vi "nanocal -- nuclear schottky fit V8.vi"() -> ()   [LabVIEW 2021] (continued)
  ,  \"σlogτN\" -> 0.000000000000   ,  \"σητ1\" -> 0.000000000000   ,  \"σητS \" -> 0.000000000000   ,  \"σητN\" -> 0.000000000000    |>   , \r\"IDS0413_220525_RAW_cal__sam_\" ->   <|    \"ζ\" -> 0.044690907244   ,  \"τ1\" -> 0.013320614253   ,  \"τS\" -> 0.013760942515   ,  \"τN\" -> 0.002327045716   ,  \"τC\" -> 0.001523256988   ,  \"κ0\" -> 0.000000001960   ,  \"mm1\" -> 0.000059136229   ,  \"mm2\" -> 0.009591413737   ,  \"mm3\" -> 0.022000296296   ,  \"T\" -> 0.360000000000   ,  \"B\" -> 0.000000000000   ,  \"θ\" -> 0.000000000000   ,  \"Reoff\" -> -7142857.142857141800   ,  \"Imoff\" -> 0.000000000000   ,  \"στ1\" -> 0.002601583253   ,  \"στS\" -> 0.000378567326   ,  \"στN\" -> 0.000355149378   ,  \"τ11 \" -> 0.000000000000   ,  \"τ12\" -> 0.000000000000   ,  \"τ22\" -> 0.000000000000   ,  \"τN1\" -> 0.000000000000   ,  \"τN2\" -> 0.000000000000   ,  \"σηlogτ1 \" -> 0.000000000000   ,  \"σηlogτS\" -> 0.000000000000   ,  \"σηlogτN\" -> 0.000000000000   ,  \"σlogτ1\" -> 0.000000000000   ,  \"σlogτS\" -> 0.000000000000   ,  \"σlogτN\" -> 0.000000000000   ,  \"σητ1\" -> 0.000000000000   ,  \"σητS \" -> 0.000000000000   ,  \"σητN\" -> 0.000000000000    |>   , \r\"IDS0414_220525_RAW_cal__ref_\" ->   <|    \"ζ\" -> 0.062609276926   ,  \"τ1\" -> 0.008775091045   ,  \"τS\" -> 0.010532925062   ,  \"τN\" -> 0.001963246111   ,  \"τC\" -> 0.001185562237   ,  \"κ0\" -> 0.000000002220   ,  \"mm1\" -> 0.000063480840   ,  \"mm2\" -> 0.006468821738   ,  \"mm3\" -> 0.016706898118   ,  \"T\" -> 0.430000000000   ,  \"B\" -> 0.000000000000   ,  \"θ\" -> 0.000000000000   ,  \"Reoff\" -> -7657142.857142858210   ,  \"Imoff\" -> 0.000000000000   ,  \"στ1\" -> 0.001587412963   ,  \"στS\" -> 0.001748149515   ,  \"στN\" -> 0.000451539809   ,  \"τ11 \" -> 0.000000000000   ,  \"τ12\" -> 0.000000000000   ,  \"τ22\" -> 0.000000000000   ,  \"τN1\" -> 0.000000000000   ,  \"τN2\" -> 0.000000000000   ,  \"σηlogτ1 \" -> 0.000000000000   ,  \"σηlogτS\" -> 0.000000000000   ,  \"σηlogτN\" -> 0.000000000000   ,  \"σlogτ1\" -> 0.000000000000   ,  \"σlogτS\" -> 0.000000000000   ,  \"σlogτN\" -> 0.000000000000   ,  \"σητ1\" -> 0.000000000000   ,  \"σητS \" -> 0.000000000000   ,  \"σητN\" -> 0.000000000000    |>   , \r\"IDS0414_220525_RAW_cal__sam_\" ->   <|    \"ζ\" -> 0.036206503728   ,  \"τ1\" -> 0.010323598347   ,  \"τS\" -> 0.013793333734   ,  \"τN\" -> 0.001947462554   ,  \"τC\" -> 0.001576858934   ,  \"κ0\" -> 0.000000002450   ,  \"mm1\" -> 0.000049775806   ,  \"mm2\" -> 0.008169881573   ,  \"mm3\" -> 0.019991515390   ,  \"T\" -> 0.430000000000   ,  \"B\" -> 0.000000000000   ,  \"θ\" -> 0.000000000000   ,  \"Reoff\" -> -5183673.469387754800   ,  \"Imoff\" -> 0.000000000000   ,  \"στ1\" -> 0.000547128250   ,  \"στS\" -> 0.000218959699   ,  \"στN\" -> 0.000102085685   ,  \"τ11 \" -> 0.000000000000   ,  \"τ12\" -> 0.000000000000   ,  \"τ22\" -> 0.000000000000   ,  \"τN1\" -> 0.000000000000   ,  \"τN2\" -> 0.000000000000   ,  \"σηlogτ1 \" -> 0.000000000000   ,  \"σηlogτS\" -> 0.000000000000   ,  \"σηlogτN\" -> 0.000000000000   ,  \"σlogτ1\" -> 0.000000000000   ,  \"σlogτS\" -> 0.000000000000   ,  \"σlogτN\" -> 0.000000000000   ,  \"σητ1\" -> 0.000000000000   ,  \"σητS \" -> 0.000000000000   ,  \"σητN\" -> 0.000000000000    |>   , \r\"IDS0415_220525_RAW_cal__ref_\" ->   <|    \"ζ\" -> 0.048185231284   ,  \"τ1\" -> 0.008100929282   ,  \"τS\" -> 0.011138600782   ,  \"τN\" -> 0.001553114505   ,  \"τC\" -> 0.001221442635   ,  \"κ0\" -> 0.000000002870   ,  \"mm1\" -> 0.000051029801   ,  \"mm2\" -> 0.006456930010   ,  \"mm3\" -> 0.016117680629   ,  \"T\" -> 0.530000000000   ,  \"B\" -> 0.000000000000   ,  \"θ\" -> 0.000000000000   ,  \"Reoff\" -> -5600000.000000000000   ,  \"Imoff\" -> 0.000000000000   ,  \"στ1\" -> 0.001291082516   ,  \"στS\" -> 0.001596793517   ,  \"στN\" -> 0.000325645365   ,  \"τ11 \" -> 0.000000000000   ,  \"τ12\" -> 0.000000000000   ,  \"τ22\" -> 0.000000000000   ,  \"τN1\" -> 0.000000000000   ,  \"τN2\" -> 0.000000000000   ,  \"σηlogτ1 \" -> 0.000000000000   ,  \"σηlogτS\" -> 0.000000000000   ,  \"σηlogτN\" -> 0.000000000000   ,  \"σlogτ1\" -> 0.000000000000   ,  \"σlogτS\" -> 0.000000000000   ,  \"σlogτN\" -> 0.000000000000   ,  \"σητ1\" -> 0.000000000000   ,  \"σητS \" -> 0.000000000000   ,  \"σητN\" -> 0.000000000000    |>   , \r\"IDS0415_220525_RAW_cal__sam_\" ->   <|    \"ζ\" -> 0.029049723552   ,  \"τ1\" -> 0.007716049820   ,  \"τS\" -> 0.014447051972   ,  \"τN\" -> 0.001246053989   ,  \"τC\" -> 0.001554051920   ,  \"κ0\" -> 0.000000003200   ,  \"mm1\" -> 0.000039813384   ,  \"mm2\" -> 0.006805314073   ,  \"mm3\" -> 0.018573960634   ,  \"T\" -> 0.530000000000   ,  \"B\" -> 0.000000000000   ,  \"θ\" -> 0.000000000000   ,  \"Reoff\" -> -3959183.673469387000   ,  \"Imoff\" -> 0.000000000000   ,  \"στ1\" -> 0.000764801064   ,  \"στS\" -> 0.002293201092   ,  \"στN\" -> 0.000221114317   ,  \"τ11 \" -> 0.000000000000   ,  \"τ12\" -> 0.000000000000   ,  \"τ22\" -> 0.000000000000   ,  \"τN1\" -> 0.000000000000   ,  \"τN2\" -> 0.000000000000   ,  \"σηlogτ1 \" -> 0.000000000000   ,  \"σηlogτS\" -> 0.000000000000   ,  \"σηlogτN\" -> 0.000000000000   ,  \"σlogτ1\" -> 0.000000000000   ,  \"σlogτS\" -> 0.000000000000   ,  \"σlogτN\" -> 0.000000000000   ,  \"σητ1\" -> 0.000000000000   ,  \"σητS \" -> 0.000000000000   ,  \"σητN\" -> 0.000000000000    |>   , \r\"IDS0416_220525_RAW_cal__ref_\" ->   <|    \"ζ\" -> 0.039880135587   ,  \"τ1\" -> 0.006886163932   ,  \"τS\" -> 0.012166095681   ,  \"τN\" -> 0.001127457198   ,  \"τC\" -> 0.001222704242   ,  \"κ0\" -> 0.000000003530   ,  \"mm1\" -> 0.000042889516   ,  \"mm2\" -> 0.005990891230   ,  \"mm3\" -> 0.015898788997   ,  \"T\" -> 0.630000000000   ,  \"B\" -> 0.000000000000   ,  \"θ\" -> 0.000000000000   ,  \"Reoff\" -> -4057142.857142858210   ,  \"Imoff\" -> 0.000000000000   ,  \"στ1\" -> 0.001015861741   ,  \"στS\" -> 0.001565951598   ,  \"στN\" -> 0.000225145356   ,  \"τ11 \" -> 0.000000000000   ,  \"τ12\" -> 0.000000000000   ,  \"τ22\" -> 0.000000000000   ,  \"τN1\" -> 0.000000000000   ,  \"τN2\" -> 0.000000000000   ,  \"σηlogτ1 \" -> 0.000000000000   ,  \"σηlogτS\" -> 0.000000000000   ,  \"σηlogτN\" -> 0.000000000000   ,  \"σlogτ1\" -> 0.000000000000   ,  \"σlogτS\" -> 0.000000000000   ,  \"σlogτN\" -> 0.000000000000   ,  \"σητ1\" -> 0.000000000000   ,  \"σητS \" -> 0.000000000000   ,  \"σητN\" -> 0.000000000000    |>   , \r\"IDS0416_220525_RAW_cal__sam_\" ->   <|    \"ζ\" -> 0.022998692784   ,  \"τ1\" -> 0.007393021158   ,  \"τS\" -> 0.015620230500   ,  \"τN\" -> 0.001040733682   ,  \"τC\" -> 0.001765774011   ,  \"κ0\" -> 0.000000003911   ,  \"mm1\" -> 0.000035818495   ,  \"mm2\" -> 0.006739334009   ,  \"mm3\" -> 0.019427787243   ,  \"T\" -> 0.630000000000   ,  \"B\" -> 0.000000000000   ,  \"θ\" -> 0.000000000000   ,  \"Reoff\" -> -2408163.265306121670   ,  \"Imoff\" -> 0.000000000000   ,  \"στ1\" -> 0.000980763421   ,  \"στS\" -> 0.002016923628   ,  \"στN\" -> 0.000219391445   ,  \"τ11 \" -> 0.000000000000   ,  \"τ12\" -> 0.000000000000   ,  \"τ22\" -> 0.000000000000   ,  \"τN1\" -> 0.000000000000   ,  \"τN2\" -> 0.000000000000   ,  \"σηlogτ1 \" -> 0.000000000000   ,  \"σηlogτS\" -> 0.000000000000   ,  \"σηlogτN\" -> 0.000000000000   ,  \"σlogτ1\" -> 0.000000000000   ,  \"σlogτS\" -> 0.000000000000   ,  \"σlogτN\" -> 0.000000000000   ,  \"σητ1\" -> 0.000000000000   ,  \"σητS \" -> 0.000000000000   ,  \"σητN\" -> 0.000000000000    |>   , \r\"IDS0417_220525_RAW_cal__ref_\" ->   <|    \"ζ\" -> 0.032750219175   ,  \"τ1\" -> 0.005623693280   ,  \"τS\" -> 0.015325743160   ,  \"τN\" -> 0.000717738154   ,  \"τC\" -> 0.001196295790   ,  \"κ0\" -> 0.000000004900   ,  \"mm1\" -> 0.000035343333   ,  \"mm2\" -> 0.005288786846   ,  \"mm3\" -> 0.018064767734   ,  \"T\" -> 0.830000000000   ,  \"B\" -> 0.000000000000   ,  \"θ\" -> 0.000000000000   ,  \"Reoff\" -> -3028571.428571429100   ,  \"Imoff\" -> 0.000000000000   ,  \"στ1\" -> 0.003777268036   ,  \"στS\" -> 0.001674973783   ,  \"στN\" -> 0.000298996570   ,  \"τ11 \" -> 0.000000000000   ,  \"τ12\" -> 0.000000000000   ,  \"τ22\" -> 0.000000000000   ,  \"τN1\" -> 0.000000000000   ,  \"τN2\" -> 0.000000000000   ,  \"σηlogτ1 \" -> 0.000000000000   ,  \"σηlogτS\" -> 0.000000000000   ,  \"σηlogτN\" -> 0.000000000000   ,  \"σlogτ1\" -> 0.000000000000   ,  \"σlogτS\" -> 0.000000000000   ,  \"σlogτN\" -> 0.000000000000   ,  \"σητ1\" -> 0.000000000000   ,  \"σητS \" -> 0.000000000000   ,  \"σητN\" -> 0.000000000000    |>   , \r\"IDS0417_220525_RAW_cal__sam_\" ->   <|    \"ζ\" -> 0.020422056832   ,  \"τ1\" -> 0.006457484957   ,  \"τS\" -> 0.019722165301   ,  \"τN\" -> 0.000729413719   ,  \"τC\" -> 0.001622930071   ,  \"κ0\" -> 0.000000005380   ,  \"mm1\" -> 0.000030097695   ,  \"mm2\" -> 0.006162713408   ,  \"mm3\" -> 0.022756846254   ,  \"T\" -> 0.830000000000   ,  \"B\" -> 0.000000000000   ,  \"θ\" -> 0.000000000000   ,  \"Reoff\" -> -2081632.653061224150   ,  \"Imoff\" -> 0.000000000000   ,  \"στ1\" -> 0.000977899540   ,  \"στS\" -> 0.002370947727   ,  \"στN\" -> 0.000160479256   ,  \"τ11 \" -> 0.000000000000   ,  \"τ12\" -> 0.000000000000   ,  \"τ22\" -> 0.000000000000   ,  \"τN1\" -> 0.000000000000   ,  \"τN2\" -> 0.000000000000   ,  \"σηlogτ1 \" -> 0.000000000000   ,  \"σηlogτS\" -> 0.000000000000   ,  \"σηlogτN\" -> 0.000000000000   ,  \"σlogτ1\" -> 0.000000000000   ,  \"σlogτS\" -> 0.000000000000   ,  \"σlogτN\" -> 0.000000000000   ,  \"σητ1\" -> 0.000000000000   ,  \"σητS \" -> 0.000000000000   ,  \"σητN\" -> 0.000000000000    |>   , \r\"IDS0418_220525_RAW_cal__ref_\" ->   <|    \"ζ\" -> 0.022904137166   ,  \"τ1\" -> 0.004842430213   ,  \"τS\" -> 0.021231337399   ,  \"τN\" -> 0.000595878691   ,  \"τC\" -> 0.001701256533   ,  \"κ0\" -> 0.000000006850   ,  \"mm1\" -> 0.000035378969   ,  \"mm2\" -> 0.004689611444   ,  \"mm3\" -> 0.024145845974   ,  \"T\" -> 1.120000000000   ,  \"B\" -> 0.000000000000   ,  \"θ\" -> 0.000000000000   ,  \"Reoff\" -> -1314285.714285716420   ,  \"Imoff\" -> 0.000000000000   ,  \"στ1\" -> 0.000594455147   ,  \"στS\" -> 0.001847173468   ,  \"στN\" -> 0.000101337306   ,  \"τ11 \" -> 0.000000000000   ,  \"τ12\" -> 0.000000000000   ,  \"τ22\" -> 0.000000000000   ,  \"τN1\" -> 0.000000000000   ,  \"τN2\" -> 0.000000000000   ,  \"σηlogτ1 \" -> 0.000000000000   ,  \"σηlogτS\" -> 0.000000000000   ,  \"σηlogτN\" -> 0.000000000000   ,  \"σlogτ1\" -> 0.000000000000   ,  \"σlogτS\" -> 0.000000000000   ,  \"σlogτN\" -> 0.000000000000   ,  \"σητ1\" -> 0.000000000000   ,  \"σητS \" -> 0.000000000000   ,  \"σητN\" -> 0.000000000000    |>   , \r\"IDS0418_220525_RAW_cal__sam_\" ->   <|    \"ζ\" -> 0.010833914814   ,  \"τ1\" -> 0.006105280968   ,  \"τS\" -> 0.027771405990   ,  \"τN\" -> 0.000655710517   ,  \"τC\" -> 0.001898693697   ,  \"κ0\" -> 0.000000007420   ,  \"mm1\" -> 0.000019072683   ,  \"mm2\" -> 0.005941306089   ,  \"mm3\" -> 0.030778689359   ,  \"T\" -> 1.120000000000   ,  \"B\" -> 0.000000000000   ,  \"θ\" -> 0.000000000000   ,  \"Reoff\" -> -608163.265306122367   ,  \"Imoff\" -> 0.000000000000   ,  \"στ1\" -> 0.001326459237   ,  \"στS\" -> 0.003728359065   ,  \"στN\" -> 0.000181682896   ,  \"τ11 \" -> 0.000000000000   ,  \"τ12\" -> 0.000000000000   ,  \"τ22\" -> 0.000000000000   ,  \"τN1\" -> 0.000000000000   ,  \"τN2\" -> 0.000000000000   ,  \"σηlogτ1 \" -> 0.000000000000   ,  \"σηlogτS\" -> 0.000000000000   ,  \"σηlogτN\" -> 0.000000000000   ,  \"σlogτ1\" -> 0.000000000000   ,  \"σlogτS\" -> 0.000000000000   ,  \"σlogτN\" -> 0.000000000000   ,  \"σητ1\" -> 0.000000000000   ,  \"σητS \" -> 0.000000000000   ,  \"σητN\" -> 0.000000000000    |>   , \r\"IDS0419_220525_RAW_cal__ref_\" ->   <|    \"ζ\" -> 0.019588015905   ,  \"τ1\" -> 0.004781626559   ,  \"τS\" -> 0.047742438651   ,  \"τN\" -> 0.000600848305   ,  \"τC\" -> 0.002316865749   ,  \"κ0\" -> 0.000000012200   ,  \"mm1\" -> 0.000042523875   ,  \"mm2\" -> 0.004719121437   ,  \"mm3\" -> 0.051627083026   ,  \"T\" -> 1.900000000000   ,  \"B\" -> 0.000000000000   ,  \"θ\" -> 0.000000000000   ,  \"Reoff\" -> -714285.714285716413   ,  \"Imoff\" -> 0.000000000000   ,  \"στ1\" -> 0.001059318885   ,  \"στS\" -> 0.005613918235   ,  \"στN\" -> 0.000174681152   ,  \"τ11 \" -> 0.000000000000   ,  \"τ12\" -> 0.000000000000   ,  \"τ22\" -> 0.000000000000   ,  \"τN1\" -> 0.000000000000   ,  \"τN2\" -> 0.000000000000   ,  \"σηlogτ1 \" -> 0.000000000000   ,  \"σηlogτS\" -> 0.000000000000   ,  \"σηlogτN\" -> 0.000000000000   ,  \"σlogτ1\" -> 0.000000000000   ,  \"σlogτS\" -> 0.000000000000   ,  \"σlogτN\" -> 0.000000000000   ,  \"σητ1\" -> 0.000000000000   ,  \"σητS \" -> 0.000000000000   ,  \"σητN\" -> 0.000000000000    |>   , \r\"IDS0419_220525_RAW_cal__sam_\" ->   <|    \"ζ\" -> 0.011595776290   ,  \"τ1\" -> 0.006117918264   ,  \"τS\" -> 0.061916055974   ,  \"τN\" -> 0.000669101537   ,  \"τC\" -> 0.002022450323   ,  \"κ0\" -> 0.000000012950   ,  \"mm1\" -> 0.000022465670   ,  \"mm2\" -> 0.006048051710   ,  \"mm3\" -> 0.065380732203   ,  \"T\" -> 1.900000000000   ,  \"B\" -> 0.000000000000   ,  \"θ\" -> 0.000000000000   ,  \"Reoff\" -> -608163.265306122367   ,  \"Imoff\" -> 0.000000000000   ,  \"στ1\" -> 0.001547930555   ,  \"στS\" -> 0.007827805463   ,  \"στN\" -> 0.000227173092   ,  \"τ11 \" -> 0.000000000000   ,  \"τ12\" -> 0.000000000000   ,  \"τ22\" -> 0.000000000000   ,  \"τN1\" -> 0.000000000000   ,  \"τN2\" -> 0.000000000000   ,  \"σηlogτ1 \" -> 0.000000000000   ,  \"σηlogτS\" -> 0.000000000000   ,  \"σηlogτN\" -> 0.000000000000   ,  \"σlogτ1\" -> 0.000000000000   ,  \"σlogτS\" -> 0.000000000000   ,  \"σlogτN\" -> 0.000000000000   ,  \"σητ1\" -> 0.000000000000   ,  \"σητS \" -> 0.000000000000   ,  \"σητN\" -> 0.000000000000    |>   , \r\"IDS0420_220525_RAW_cal__ref_\" ->   <|    \"ζ\" -> 0.020834428044   ,  \"τ1\" -> 0.004699063518   ,  \"τS\" -> 0.052089260804   ,  \"τN\" -> 0.000594934592   ,  \"τC\" -> 0.002174562230   ,  \"κ0\" -> 0.000000013800   ,  \"mm1\" -> 0.000042670178   ,  \"mm2\" -> 0.004643420551   ,  \"mm3\" -> 0.055969375493   ,  \"T\" -> 2.100000000000   ,  \"B\" -> 0.000000000000   ,  \"θ\" -> 0.000000000000   ,  \"Reoff\" -> -714285.714285716413   ,  \"Imoff\" -> 0.000000000000   ,  \"στ1\" -> 0.001320131062   ,  \"στS\" -> 0.004774189877   ,  \"στN\" -> 0.000170930701   ,  \"τ11 \" -> 0.000000000000   ,  \"τ12\" -> 0.000000000000   ,  \"τ22\" -> 0.000000000000   ,  \"τN1\" -> 0.000000000000   ,  \"τN2\" -> 0.000000000000   ,  \"σηlogτ1 \" -> 0.000000000000   ,  \"σηlogτS\" -> 0.000000000000   ,  \"σηlogτN\" -> 0.000000000000   ,  \"σlogτ1\" -> 0.000000000000   ,  \"σlogτS\" -> 0.000000000000   ,  \"σlogτN\" -> 0.000000000000   ,  \"σητ1\" -> 0.000000000000   ,  \"σητS \" -> 0.000000000000   ,  \"σητN\" -> 0.000000000000    |>   , \r\"IDS0420_220525_RAW_cal__sam_\" ->   <|    \"ζ\" -> 0.011850996022   ,  \"τ1\" -> 0.005764384736   ,  \"τS\" -> 0.066220067505   ,  \"τN\" -> 0.000645440877   ,  \"τC\" -> 0.002901198812   ,  \"κ0\" -> 0.000000014700   ,  \"mm1\" -> 0.000032584327   ,  \"mm2\" -> 0.005706320364   ,  \"mm3\" -> 0.070584610113   ,  \"T\" -> 2.100000000000   ,  \"B\" -> 0.000000000000   ,  \"θ\" -> 0.000000000000   ,  \"Reoff\" -> -461224.489795918343   ,  \"Imoff\" -> 0.000000000000   ,  \"στ1\" -> 0.000879947943   ,  \"στS\" -> 0.005816006372   ,  \"στN\" -> 0.000150645668   ,  \"τ11 \" -> 0.000000000000   ,  \"τ12\" -> 0.000000000000   ,  \"τ22\" -> 0.000000000000   ,  \"τN1\" -> 0.000000000000   ,  \"τN2\" -> 0.000000000000   ,  \"σηlogτ1 \" -> 0.000000000000   ,  \"σηlogτS\" -> 0.000000000000   ,  \"σηlogτN\" -> 0.000000000000   ,  \"σlogτ1\" -> 0.000000000000   ,  \"σlogτS\" -> 0.000000000000   ,  \"σlogτN\" -> 0.000000000000   ,  \"σητ1\" -> 0.000000000000   ,  \"σητS \" -> 0.000000000000   ,  \"σητN\" -> 0.000000000000    |>   , \r\"IDS0421_220525_RAW_cal__ref_\" ->   <|    \"ζ\" -> 0.022335092396   ,  \"τ1\" -> 0.004357676744   ,  \"τS\" -> 0.014734142286   ,  \"τN\" -> 0.000494755663   ,  \"τC\" -> 0.002291218216   ,  \"κ0\" -> 0.000000015200   ,  \"mm1\" -> 0.000043555244   ,  \"mm2\" -> 0.004196096690   ,  \"mm3\" -> 0.017978279817   ,  \"T\" -> 2.300000000000   ,  \"B\" -> 0.000000000000   ,  \"θ\" -> 0.000000000000   ,  \"Reoff\" -> -714285.714285716413   ,  \"Imoff\" -> 0.000000000000   ,  \"στ1\" -> 0.001017327919   ,  \"στS\" -> 0.002314643379   ,  \"στN\" -> 0.000146182526   ,  \"τ11 \" -> 0.000000000000   ,  \"τ12\" -> 0.000000000000   ,  \"τ22\" -> 0.000000000000   ,  \"τN1\" -> 0.000000000000   ,  \"τN2\" -> 0.000000000000   ,  \"σηlogτ1 \" -> 0.000000000000   ,  \"σηlogτS\" -> 0.000000000000   ,  \"σηlogτN\" -> 0.000000000000   ,  \"σlogτ1\" -> 0.000000000000   ,  \"σlogτS\" -> 0.000000000000   ,  \"σlogτN\" -> 0.000000000000   ,  \"σητ1\" -> 0.000000000000   ,  \"σητS \" -> 0.000000000000   ,  \"σητN\" -> 0.000000000000    |>   , \r\"IDS0421_220525_RAW_cal__sam_\" ->   <|    \"ζ\" -> 0.017472306497   ,  \"τ1\" -> 0.005884707777   ,  \"τS\" -> 0.018273540555   ,  \"τN\" -> 0.000393530305   ,  \"τC\" -> 0.002873982576   ,  \"κ0\" -> 0.000000016000   ,  \"mm1\" -> 0.000042829990   ,  \"mm2\" -> 0.005738391469   ,  \"mm3\" -> 0.021970696537   ,  \"T\" -> 2.300000000000   ,  \"B\" -> 0.000000000000   ,  \"θ\" -> 0.000000000000   ,  \"Reoff\" -> -616326.530612244968   ,  \"Imoff\" -> 0.000000000000   ,  \"στ1\" -> 0.001449504442   ,  \"στS\" -> 0.003094967894   ,  \"στN\" -> 0.000132016087   ,  \"τ11 \" -> 0.000000000000   ,  \"τ12\" -> 0.000000000000   ,  \"τ22\" -> 0.000000000000   ,  \"τN1\" -> 0.000000000000   ,  \"τN2\" -> 0.000000000000   ,  \"σηlogτ1 \" -> 0.000000000000   ,  \"σηlogτS\" -> 0.000000000000   ,  \"σηlogτN\" -> 0.000000000000   ,  \"σlogτ1\" -> 0.000000000000   ,  \"σlogτS\" -> 0.000000000000   ,  \"σlogτN\" -> 0.000000000000   ,  \"σητ1\" -> 0.000000000000   ,  \"σητS \" -> 0.000000000000   ,  \"σητN\" -> 0.000000000000    |>   , \r\"IDS0422_220525_RAW_cal__ref_\" ->   <|    \"ζ\" -> 0.018555902016   ,  \"τ1\" -> 0.004075291246   ,  \"τS\" -> 0.009145270052   ,  \"τN\" -> 0.000208864759   ,  \"τC\" -> 0.002022167505   ,  \"κ0\" -> 0.000000022500   ,  \"mm1\" -> 0.000030348931   ,  \"mm2\" -> 0.003960776557   ,  \"mm3\" -> 0.011634042483   ,  \"T\" -> 3.100000000000   ,  \"B\" -> 0.000000000000   ,  \"θ\" -> 0.000000000000   ,  \"Reoff\" -> -371428.571428570896   ,  \"Imoff\" -> 0.000000000000   ,  \"στ1\" -> 0.000657121780   ,  \"στS\" -> 0.001216403398   ,  \"στN\" -> 0.000050486757   ,  \"τ11 \" -> 0.000000000000   ,  \"τ12\" -> 0.000000000000   ,  \"τ22\" -> 0.000000000000   ,  \"τN1\" -> 0.000000000000   ,  \"τN2\" -> 0.000000000000   ,  \"σηlogτ1 \" -> 0.000000000000   ,  \"σηlogτS\" -> 0.000000000000   ,  \"σηlogτN\" -> 0.000000000000   ,  \"σlogτ1\" -> 0.000000000000   ,  \"σlogτS\" -> 0.000000000000   ,  \"σlogτN\" -> 0.000000000000   ,  \"σητ1\" -> 0.000000000000   ,  \"σητS \" -> 0.000000000000   ,  \"σητN\" -> 0.000000000000    |>   , \r\"IDS0422_220525_RAW_cal__sam_\" ->   <|    \"ζ\" -> 0.013782660001   ,  \"τ1\" -> 0.005602489845   ,  \"τS\" -> 0.011122141420   ,  \"τN\" -> 0.000341635093   ,  \"τC\" -> 0.002887063483   ,  \"κ0\" -> 0.000000023500   ,  \"mm1\" -> 0.000031317292   ,  \"mm2\" -> 0.005389288482   ,  \"mm3\" -> 0.014690725401   ,  \"T\" -> 3.100000000000   ,  \"B\" -> 0.000000000000   ,  \"θ\" -> 0.000000000000   ,  \"Reoff\" -> -338775.510204081656   ,  \"Imoff\" -> 0.000000000000   ,  \"στ1\" -> 0.000787586702   ,  \"στS\" -> 0.001319427978   ,  \"στN\" -> 0.000072408344   ,  \"τ11 \" -> 0.000000000000   ,  \"τ12\" -> 0.000000000000   ,  \"τ22\" -> 0.000000000000   ,  \"τN1\" -> 0.000000000000   ,  \"τN2\" -> 0.000000000000   ,  \"σηlogτ1 \" -> 0.000000000000   ,  \"σηlogτS\" -> 0.000000000000   ,  \"σηlogτN\" -> 0.000000000000   ,  \"σlogτ1\" -> 0.000000000000   ,  \"σlogτS\" -> 0.000000000000   ,  \"σlogτN\" -> 0.000000000000   ,  \"σητ1\" -> 0.000000000000   ,  \"σητS \" -> 0.000000000000   ,  \"σητN\" -> 0.000000000000    |>   , \r\"IDS0424_220526_RAW_cal__ref_\" ->   <|    \"ζ\" -> 0.257512497689   ,  \"τ1\" -> 0.039924767980   ,  \"τS\" -> 0.063776955906   ,  \"τN\" -> 0.051107290948   ,  \"τC\" -> 0.000802475621   ,  \"κ0\" -> 0.000000000773   ,  \"mm1\" -> 0.000163026258   ,  \"mm2\" -> 0.019497997616   ,  \"mm3\" -> 0.165534595934   ,  \"T\" -> 0.190000000000   ,  \"B\" -> 10.000000000000   ,  \"θ\" -> 0.000000000000   ,  \"Reoff\" -> -55142857.142857134400   ,  \"Imoff\" -> 0.000000000000   ,  \"στ1\" -> 0.000058307175   ,  \"στS\" -> 0.000031998048   ,  \"στN\" -> 0.000036682192   ,  \"τ11 \" -> 0.000000000000   ,  \"τ12\" -> 0.000000000000   ,  \"τ22\" -> 0.000000000000   ,  \"τN1\" -> 0.000000000000   ,  \"τN2\" -> 0.000000000000   ,  \"σηlogτ1 \" -> 0.000000000000   ,  \"σηlogτS\" -> 0.000000000000   ,  \"σηlogτN\" -> 0.000000000000   ,  \"σlogτ1\" -> 0.000000000000   ,  \"σlogτS\" -> 0.000000000000   ,  \"σlogτN\" -> 0.000000000000   ,  \"σητ1\" -> 0.000000000000   ,  \"σητS \" -> 0.000000000000   ,  \"σητN\" -> 0.000000000000    |>   , \r\"IDS0424_220526_RAW_cal__sam_\" ->   <|    \"ζ\" -> 0.143096873941   ,  \"τ1\" -> 0.119527741552   ,  \"τS\" -> 0.213771204505   ,  \"τN\" -> 0.133065206622   ,  \"τC\" -> 0.001041786526   ,  \"κ0\" -> 0.000000000890   ,  \"mm1\" -> 0.000129929317   ,  \"mm2\" -> 0.064852834373   ,  \"mm3\" -> 0.452054381716   ,  \"T\" -> 0.190000000000   ,  \"B\" -> 10.000000000000   ,  \"θ\" -> 0.000000000000   ,  \"Reoff\" -> -41461224.489795915800   ,  \"Imoff\" -> 0.000000000000   ,  \"στ1\" -> 0.142328196867   ,  \"στS\" -> 0.153709890516   ,  \"στN\" -> 0.034979737706   ,  \"τ11 \" -> 0.000000000000   ,  \"τ12\" -> 0.000000000000   ,  \"τ22\" -> 0.000000000000   ,  \"τN1\" -> 0.000000000000   ,  \"τN2\" -> 0.000000000000   ,  \"σηlogτ1 \" -> 0.000000000000   ,  \"σηlogτS\" -> 0.000000000000   ,  \"σηlogτN\" -> 0.000000000000   ,  \"σlogτ1\" -> 0.000000000000   ,  \"σlogτS\" -> 0.000000000000   ,  \"σlogτN\" -> 0.000000000000   ,  \"σητ1\" -> 0.000000000000   ,  \"σητS \" -> 0.000000000000   ,  \"σητN\" -> 0.000000000000    |>   , \r\"IDS0425_220526_RAW_cal__ref_\" ->   <|    \"ζ\" -> 0.159335076752   ,  \"τ1\" -> 0.031885685275   ,  \"τS\" -> 0.047996731633   ,  \"τN\" -> 0.019207310502   ,  \"τC\" -> 0.000887935907   ,  \"κ0\" -> 0.000000001118   ,  \"mm1\" -> 0.000120371950   ,  \"mm2\" -> 0.019822778110   ,  \"mm3\" -> 0.090742474469   ,  \"T\" -> 0.250000000000   ,  \"B\" -> 10.000000000000   ,  \"θ\" -> 0.000000000000   ,  \"Reoff\" -> -27579558.011049721400   ,  \"Imoff\" -> 0.000000000000   ,  \"στ1\" -> 0.000105033309   ,  \"στS\" -> 0.000027614157   ,  \"στN\" -> 0.000060474658   ,  \"τ11 \" -> 0.000000000000   ,  \"τ12\" -> 0.000000000000   ,  \"τ22\" -> 0.000000000000   ,  \"τN1\" -> 0.000000000000   ,  \"τN2\" -> 0.000000000000   ,  \"σηlogτ1 \" -> 0.000000000000   ,  \"σηlogτS\" -> 0.000000000000   ,  \"σηlogτN\" -> 0.000000000000   ,  \"σlogτ1\" -> 0.000000000000   ,  \"σlogτS\" -> 0.000000000000   ,  \"σlogτN\" -> 0.000000000000   ,  \"σητ1\" -> 0.000000000000   ,  \"σητS \" -> 0.000000000000   ,  \"σητN\" -> 0.000000000000    |>   , \r\"IDS0425_220526_RAW_cal__sam_\" ->   <|    \"ζ\" -> 0.080613368975   ,  \"τ1\" -> 0.039981630615   ,  \"τS\" -> 0.067451052819   ,  \"τN\" -> 0.024952731947   ,  \"τC\" -> 0.001301901326   ,  \"κ0\" -> 0.000000001270   ,  \"mm1\" -> 0.000095538727   ,  \"mm2\" -> 0.025680137218   ,  \"mm3\" -> 0.115360621158   ,  \"T\" -> 0.250000000000   ,  \"B\" -> 10.000000000000   ,  \"θ\" -> 0.000000000000   ,  \"Reoff\" -> -15077551.020408168400   ,  \"Imoff\" -> 0.000000000000   ,  \"στ1\" -> 0.017921325903   ,  \"στS\" -> 0.008554959302   ,  \"στN\" -> 0.012696106226   ,  \"τ11 \" -> 0.000000000000   ,  \"τ12\" -> 0.000000000000   ,  \"τ22\" -> 0.000000000000   ,  \"τN1\" -> 0.000000000000   ,  \"τN2\" -> 0.000000000000   ,  \"σηlogτ1 \" -> 0.000000000000   ,  \"σηlogτS\" -> 0.000000000000   ,  \"σηlogτN\" -> 0.000000000000   ,  \"σlogτ1\" -> 0.000000000000   ,  \"σlogτS\" -> 0.000000000000   ,  \"σlogτN\" -> 0.000000000000   ,  \"σητ1\" -> 0.000000000000   ,  \"σητS \" -> 0.000000000000   ,  \"σητN\" -> 0.000000000000    |>   , \r\"IDS0426_220526_RAW_cal__ref_\" ->   <|    \"ζ\" -> 0.111460827005   ,  \"τ1\" -> 0.024224453348   ,  \"τS\" -> 0.042028783084   ,  \"τN\" -> 0.009416687783   ,  \"τC\" -> 0.001053496592   ,  \"κ0\" -> 0.000000001428   ,  \"mm1\" -> 0.000103540379   ,  \"mm2\" -> 0.017919606240   ,  \"mm3\" -> 0.064434428916   ,  \"T\" -> 0.300000000000   ,  \"B\" -> 10.000000000000   ,  \"θ\" -> 0.000000000000   ,  \"Reoff\" -> -13408163.265306122600   ,  \"Imoff\" -> 0.000000000000   ,  \"στ1\" -> 0.000203310758   ,  \"στS\" -> 0.000031022481   ,  \"στN\" -> 0.000119793909   ,  \"τ11 \" -> 0.000000000000   ,  \"τ12\" -> 0.000000000000   ,  \"τ22\" -> 0.000000000000   ,  \"τN1\" -> 0.000000000000   ,  \"τN2\" -> 0.000000000000   ,  \"σηlogτ1 \" -> 0.000000000000   ,  \"σηlogτS\" -> 0.000000000000   ,  \"σηlogτN\" -> 0.000000000000   ,  \"σlogτ1\" -> 0.000000000000   ,  \"σlogτS\" -> 0.000000000000   ,  \"σlogτN\" -> 0.000000000000   ,  \"σητ1\" -> 0.000000000000   ,  \"σητS \" -> 0.000000000000   ,  \"σητN\" -> 0.000000000000    |>   , \r\"IDS0426_220526_RAW_cal__sam_\" ->   <|    \"ζ\" -> 0.000000000000   ,  \"τ1\" -> 0.000000000000   ,  \"τS\" -> 0.000000000000   ,  \"τN\" -> 0.000000000000   ,  \"τC\" -> 0.000000000000   ,  \"κ0\" -> 0.000000000000   ,  \"mm1\" -> 0.000000000000   ,  \"mm2\" -> 0.000000000000   ,  \"mm3\" -> 0.000000000000   ,  \"T\" -> 0.300000000000   ,  \"B\" -> 10.000000000000   ,  \"θ\" -> 0.000000000000   ,  \"Reoff\" -> 0.000000000000   ,  \"Imoff\" -> 0.000000000000   ,  \"στ1\" -> 0.000000000000   ,  \"στS\" -> 0.000000000000   ,  \"στN\" -> 0.000000000000   ,  \"τ11 \" -> 0.000000000000   ,  \"τ12\" -> 0.000000000000   ,  \"τ22\" -> 0.000000000000   ,  \"τN1\" -> 0.000000000000   ,  \"τN2\" -> 0.000000000000   ,  \"σηlogτ1 \" -> 0.000000000000   ,  \"σηlogτS\" -> 0.000000000000   ,  \"σηlogτN\" -> 0.000000000000   ,  \"σlogτ1\" -> 0.000000000000   ,  \"σlogτS\" -> 0.000000000000   ,  \"σlogτN\" -> 0.000000000000   ,  \"σητ1\" -> 0.000000000000   ,  \"σητS \" -> 0.000000000000   ,  \"σητN\" -> 0.000000000000    |>   , \r\"IDS0427_220526_RAW_cal__ref_\" ->   <|    \"ζ\" -> 0.410372558234   ,  \"τ1\" -> 0.044042677076   ,  \"τS\" -> 0.102926494068   ,  \"τN\" -> 0.135379226142   ,  \"τC\" -> 0.000829804272   ,  \"κ0\" -> 0.000000000538   ,  \"mm1\" -> 0.000240462729   ,  \"mm2\" -> 0.017682403463   ,  \"mm3\" -> 0.363049463410   ,  \"T\" -> 0.150000000000   ,  \"B\" -> 10.000000000000   ,  \"θ\" -> 0.000000000000   ,  \"Reoff\" -> -106571428.571428567000   ,  \"Imoff\" -> 0.000000000000   ,  \"στ1\" -> 0.000056157157   ,  \"στS\" -> 0.000057678080   ,  \"στN\" -> 0.000041998406   ,  \"τ11 \" -> 0.000000000000   ,  \"τ12\" -> 0.000000000000   ,  \"τ22\" -> 0.000000000000   ,  \"τN1\" -> 0.000000000000   ,  \"τN2\" -> 0.000000000000   ,  \"σηlogτ1 \" -> 0.000000000000   ,  \"σηlogτS\" -> 0.000000000000   ,  \"σηlogτN\" -> 0.000000000000   ,  \"σlogτ1\" -> 0.000000000000   ,  \"σlogτS\" -> 0.000000000000   ,  \"σlogτN\" -> 0.000000000000   ,  \"σητ1\" -> 0.000000000000   ,  \"σητS \" -> 0.000000000000   ,  \"σητN\" -> 0.000000000000    |>   , \r\"IDS0427_220526_RAW_cal__sam_\" ->   <|    \"ζ\" -> 0.000000000000   ,  \"τ1\" -> 0.000000000000   ,  \"τS\" -> 0.000000000000   ,  \"τN\" -> 0.000000000000   ,  \"τC\" -> 0.000000000000   ,  \"κ0\" -> 0.000000000000   ,  \"mm1\" -> 0.000000000000   ,  \"mm2\" -> 0.000000000000   ,  \"mm3\" -> 0.000000000000   ,  \"T\" -> 0.150000000000   ,  \"B\" -> 10.000000000000   ,  \"θ\" -> 0.000000000000   ,  \"Reoff\" -> 0.000000000000   ,  \"Imoff\" -> 0.000000000000   ,  \"στ1\" -> 0.000000000000   ,  \"στS\" -> 0.000000000000   ,  \"στN\" -> 0.000000000000   ,  \"τ11 \" -> 0.000000000000   ,  \"τ12\" -> 0.000000000000   ,  \"τ22\" -> 0.000000000000   ,  \"τN1\" -> 0.000000000000   ,  \"τN2\" -> 0.000000000000   ,  \"σηlogτ1 \" -> 0.000000000000   ,  \"σηlogτS\" -> 0.000000000000   ,  \"σηlogτN\" -> 0.000000000000   ,  \"σlogτ1\" -> 0.000000000000   ,  \"σlogτS\" -> 0.000000000000   ,  \"σlogτN\" -> 0.000000000000   ,  \"σητ1\" -> 0.000000000000   ,  \"σητS \" -> 0.000000000000   ,  \"σητN\" -> 0.000000000000    |>   , \r\"IDS0428_220526_RAW_cal__ref_\" ->   <|    \"ζ\" -> 0.085761087931   ,  \"τ1\" -> 0.025055116447   ,  \"τS\" -> 0.039037181879   ,  \"τN\" -> 0.005587062279   ,  \"τC\" -> 0.001009401057   ,  \"κ0\" -> 0.000000001845   ,  \"mm1\" -> 0.000078014543   ,  \"mm2\" -> 0.019900208864   ,  \"mm3\" -> 0.054537561983   ,  \"T\" -> 0.360000000000   ,  \"B\" -> 10.000000000000   ,  \"θ\" -> 0.000000000000   ,  \"Reoff\" -> -10418232.044198893000   ,  \"Imoff\" -> 0.000000000000   ,  \"στ1\" -> 0.000347384848   ,  \"στS\" -> 0.000031989956   ,  \"στN\" -> 0.000188370043   ,  \"τ11 \" -> 0.000000000000   ,  \"τ12\" -> 0.000000000000   ,  \"τ22\" -> 0.000000000000   ,  \"τN1\" -> 0.000000000000   ,  \"τN2\" -> 0.000000000000   ,  \"σηlogτ1 \" -> 0.000000000000   ,  \"σηlogτS\" -> 0.000000000000   ,  \"σηlogτN\" -> 0.000000000000   ,  \"σlogτ1\" -> 0.000000000000   ,  \"σlogτS\" -> 0.000000000000   ,  \"σlogτN\" -> 0.000000000000   ,  \"σητ1\" -> 0.000000000000   ,  \"σητS \" -> 0.000000000000   ,  \"σητN\" -> 0.000000000000    |>   , \r\"IDS0428_220526_RAW_cal__sam_\" ->   <|    \"ζ\" -> 0.000000000000   ,  \"τ1\" -> 0.000000000000   ,  \"τS\" -> 0.000000000000   ,  \"τN\" -> 0.000000000000   ,  \"τC\" -> 0.000000000000   ,  \"κ0\" -> 0.000000000000   ,  \"mm1\" -> 0.000000000000   ,  \"mm2\" -> 0.000000000000   ,  \"mm3\" -> 0.000000000000   ,  \"T\" -> 0.360000000000   ,  \"B\" -> 10.000000000000   ,  \"θ\" -> 0.000000000000   ,  \"Reoff\" -> 0.000000000000   ,  \"Imoff\" -> 0.000000000000   ,  \"στ1\" -> 0.000000000000   ,  \"στS\" -> 0.000000000000   ,  \"στN\" -> 0.000000000000   ,  \"τ11 \" -> 0.000000000000   ,  \"τ12\" -> 0.000000000000   ,  \"τ22\" -> 0.000000000000   ,  \"τN1\" -> 0.000000000000   ,  \"τN2\" -> 0.000000000000   ,  \"σηlogτ1 \" -> 0.000000000000   ,  \"σηlogτS\" -> 0.000000000000   ,  \"σηlogτN\" -> 0.000000000000   ,  \"σlogτ1\" -> 0.000000000000   ,  \"σlogτS\" -> 0.000000000000   ,  \"σlogτN\" -> 0.000000000000   ,  \"σητ1\" -> 0.000000000000   ,  \"σητS \" -> 0.000000000000   ,  \"σητN\" -> 0.000000000000    |>   , \r\"IDS0429_220526_RAW_cal__ref_\" ->   <|    \"ζ\" -> 0.061793425944   ,  \"τ1\" -> 0.022729976964   ,  \"τS\" -> 0.037992561842   ,  \"τN\" -> 0.003473638845   ,  \"τC\" -> 0.001146343524   ,  \"κ0\" -> 0.000000002261   ,  \"mm1\" -> 0.000064971896   ,  \"mm2\" -> 0.019461604024   ,  \"mm3\" -> 0.048378283857   ,  \"T\" -> 0.420000000000   ,  \"B\" -> 10.000000000000   ,  \"θ\" -> 0.000000000000   ,  \"Reoff\" -> -5435911.602209940560   ,  \"Imoff\" -> 0.000000000000   ,  \"στ1\" -> 0.000628479456   ,  \"στS\" -> 0.000037704094   ,  \"στN\" -> 0.000344539444   ,  \"τ11 \" -> 0.000000000000   ,  \"τ12\" -> 0.000000000000   ,  \"τ22\" -> 0.000000000000   ,  \"τN1\" -> 0.000000000000   ,  \"τN2\" -> 0.000000000000   ,  \"σηlogτ1 \" -> 0.000000000000   ,  \"σηlogτS\" -> 0.000000000000   ,  \"σηlogτN\" -> 0.000000000000   ,  \"σlogτ1\" -> 0.000000000000   ,  \"σlogτS\" -> 0.000000000000   ,  \"σlogτN\" -> 0.000000000000   ,  \"σητ1\" -> 0.000000000000   ,  \"σητS \" -> 0.000000000000   ,  \"σητN\" -> 0.000000000000    |>   , \r\"IDS0429_220526_RAW_cal__sam_\" ->   <|    \"ζ\" -> 0.000000000000   ,  \"τ1\" -> 0.000000000000   ,  \"τS\" -> 0.000000000000   ,  \"τN\" -> 0.000000000000   ,  \"τC\" -> 0.000000000000   ,  \"κ0\" -> 0.000000000000   ,  \"mm1\" -> 0.000000000000   ,  \"mm2\" -> 0.000000000000   ,  \"mm3\" -> 0.000000000000   ,  \"T\" -> 0.420000000000   ,  \"B\" -> 10.000000000000   ,  \"θ\" -> 0.000000000000   ,  \"Reoff\" -> 0.000000000000   ,  \"Imoff\" -> 0.000000000000   ,  \"στ1\" -> 0.000000000000   ,  \"στS\" -> 0.000000000000   ,  \"στN\" -> 0.000000000000   ,  \"τ11 \" -> 0.000000000000   ,  \"τ12\" -> 0.000000000000   ,  \"τ22\" -> 0.000000000000   ,  \"τN1\" -> 0.000000000000   ,  \"τN2\" -> 0.000000000000   ,  \"σηlogτ1 \" -> 0.000000000000   ,  \"σηlogτS\" -> 0.000000000000   ,  \"σηlogτN\" -> 0.000000000000   ,  \"σlogτ1\" -> 0.000000000000   ,  \"σlogτS\" -> 0.000000000000   ,  \"σlogτN\" -> 0.000000000000   ,  \"σητ1\" -> 0.000000000000   ,  \"σητS \" -> 0.000000000000   ,  \"σητN\" -> 0.000000000000    |>   , \r\"IDS0430_220526_RAW_cal__ref_\" ->   <|    \"ζ\" -> 0.045410527771   ,  \"τ1\" -> 0.022224368069   ,  \"τS\" -> 0.038327267568   ,  \"τN\" -> 0.002127889601   ,  \"τC\" -> 0.001500583676   ,  \"κ0\" -> 0.000000002914   ,  \"mm1\" -> 0.000062924210   ,  \"mm2\" -> 0.020129743814   ,  \"mm3\" -> 0.045824530928   ,  \"T\" -> 0.520000000000   ,  \"B\" -> 10.000000000000   ,  \"θ\" -> 0.000000000000   ,  \"Reoff\" -> -3224489.795918375260   ,  \"Imoff\" -> 0.000000000000   ,  \"στ1\" -> 0.001280571461   ,  \"στS\" -> 0.000046989648   ,  \"στN\" -> 0.000705007313   ,  \"τ11 \" -> 0.000000000000   ,  \"τ12\" -> 0.000000000000   ,  \"τ22\" -> 0.000000000000   ,  \"τN1\" -> 0.000000000000   ,  \"τN2\" -> 0.000000000000   ,  \"σηlogτ1 \" -> 0.000000000000   ,  \"σηlogτS\" -> 0.000000000000   ,  \"σηlogτN\" -> 0.000000000000   ,  \"σlogτ1\" -> 0.000000000000   ,  \"σlogτS\" -> 0.000000000000   ,  \"σlogτN\" -> 0.000000000000   ,  \"σητ1\" -> 0.000000000000   ,  \"σητS \" -> 0.000000000000   ,  \"σητN\" -> 0.000000000000    |>   , \r\"IDS0430_220526_RAW_cal__sam_\" ->   <|    \"ζ\" -> 0.000000000000   ,  \"τ1\" -> 0.000000000000   ,  \"τS\" -> 0.000000000000   ,  \"τN\" -> 0.000000000000   ,  \"τC\" -> 0.000000000000   ,  \"κ0\" -> 0.000000000000   ,  \"mm1\" -> 0.000000000000   ,  \"mm2\" -> 0.000000000000   ,  \"mm3\" -> 0.000000000000   ,  \"T\" -> 0.520000000000   ,  \"B\" -> 10.000000000000   ,  \"θ\" -> 0.000000000000   ,  \"Reoff\" -> 0.000000000000   ,  \"Imoff\" -> 0.000000000000   ,  \"στ1\" -> 0.000000000000   ,  \"στS\" -> 0.000000000000   ,  \"στN\" -> 0.000000000000   ,  \"τ11 \" -> 0.000000000000   ,  \"τ12\" -> 0.000000000000   ,  \"τ22\" -> 0.000000000000   ,  \"τN1\" -> 0.000000000000   ,  \"τN2\" -> 0.000000000000   ,  \"σηlogτ1 \" -> 0.000000000000   ,  \"σηlogτS\" -> 0.000000000000   ,  \"σηlogτN\" -> 0.000000000000   ,  \"σlogτ1\" -> 0.000000000000   ,  \"σlogτS\" -> 0.000000000000   ,  \"σlogτN\" -> 0.000000000000   ,  \"σητ1\" -> 0.000000000000   ,  \"σητS \" -> 0.000000000000   ,  \"σητN\" -> 0.000000000000    |>   , \r\"IDS0431_220527_RAW_cal__ref_\" ->   <|    \"ζ\" -> 0.587332924785   ,  \"τ1\" -> 0.048285770693   ,  \"τS\" -> 0.172123299088   ,  \"τN\" -> 0.328986383817   ,  \"τC\" -> 0.000861567300   ,  \"κ0\" -> 0.000000000408   ,  \"mm1\" -> 0.000318149705   ,  \"mm2\" -> 0.015959319465   ,  \"mm3\" -> 0.828297767426   ,  \"T\" -> 0.120000000000   ,  \"B\" -> 10.000000000000   ,  \"θ\" -> 0.000000000000   ,  \"Reoff\" -> -187142857.142857134000   ,  \"Imoff\" -> 0.000000000000   ,  \"στ1\" -> 0.034505118075   ,  \"στS\" -> 0.052461851284   ,  \"στN\" -> 0.093268528407   ,  \"τ11 \" -> 0.000000000000   ,  \"τ12\" -> 0.000000000000   ,  \"τ22\" -> 0.000000000000   ,  \"τN1\" -> 0.000000000000   ,  \"τN2\" -> 0.000000000000   ,  \"σηlogτ1 \" -> 0.000000000000   ,  \"σηlogτS\" -> 0.000000000000   ,  \"σηlogτN\" -> 0.000000000000   ,  \"σlogτ1\" -> 0.000000000000   ,  \"σlogτS\" -> 0.000000000000   ,  \"σlogτN\" -> 0.000000000000   ,  \"σητ1\" -> 0.000000000000   ,  \"σητS \" -> 0.000000000000   ,  \"σητN\" -> 0.000000000000    |>   , \r\"IDS0431_220527_RAW_cal__sam_\" ->   <|    \"ζ\" -> 0.000000000000   ,  \"τ1\" -> 0.000000000000   ,  \"τS\" -> 0.000000000000   ,  \"τN\" -> 0.000000000000   ,  \"τC\" -> 0.000000000000   ,  \"κ0\" -> 0.000000000000   ,  \"mm1\" -> 0.000000000000   ,  \"mm2\" -> 0.000000000000   ,  \"mm3\" -> 0.000000000000   ,  \"T\" -> 0.120000000000   ,  \"B\" -> 10.000000000000   ,  \"θ\" -> 0.000000000000   ,  \"Reoff\" -> 0.000000000000   ,  \"Imoff\" -> 0.000000000000   ,  \"στ1\" -> 0.000000000000   ,  \"στS\" -> 0.000000000000   ,  \"στN\" -> 0.000000000000   ,  \"τ11 \" -> 0.000000000000   ,  \"τ12\" -> 0.000000000000   ,  \"τ22\" -> 0.000000000000   ,  \"τN1\" -> 0.000000000000   ,  \"τN2\" -> 0.000000000000   ,  \"σηlogτ1 \" -> 0.000000000000   ,  \"σηlogτS\" -> 0.000000000000   ,  \"σηlogτN\" -> 0.000000000000   ,  \"σlogτ1\" -> 0.000000000000   ,  \"σlogτS\" -> 0.000000000000   ,  \"σlogτN\" -> 0.000000000000   ,  \"σητ1\" -> 0.000000000000   ,  \"σητS \" -> 0.000000000000   ,  \"σητN\" -> 0.000000000000    |>   , \r\"IDS0432_220527_RAW_cal__ref_\" ->   <|    \"ζ\" -> 0.323198567211   ,  \"τ1\" -> 0.041879804217   ,  \"τS\" -> 0.073059196167   ,  \"τN\" -> 0.074071913735   ,  \"τC\" -> 0.000754510691   ,  \"κ0\" -> 0.000000000676   ,  \"mm1\" -> 0.000183205866   ,  \"mm2\" -> 0.018639437051   ,  \"mm3\" -> 0.218495345806   ,  \"T\" -> 0.170000000000   ,  \"B\" -> 10.000000000000   ,  \"θ\" -> 0.000000000000   ,  \"Reoff\" -> -82571428.571428567200   ,  \"Imoff\" -> 0.000000000000   ,  \"στ1\" -> 0.000050882470   ,  \"στS\" -> 0.000038008306   ,  \"στN\" -> 0.000034915711   ,  \"τ11 \" -> 0.000000000000   ,  \"τ12\" -> 0.000000000000   ,  \"τ22\" -> 0.000000000000   ,  \"τN1\" -> 0.000000000000   ,  \"τN2\" -> 0.000000000000   ,  \"σηlogτ1 \" -> 0.000000000000   ,  \"σηlogτS\" -> 0.000000000000   ,  \"σηlogτN\" -> 0.000000000000   ,  \"σlogτ1\" -> 0.000000000000   ,  \"σlogτS\" -> 0.000000000000   ,  \"σlogτN\" -> 0.000000000000   ,  \"σητ1\" -> 0.000000000000   ,  \"σητS \" -> 0.000000000000   ,  \"σητN\" -> 0.000000000000    |>   , \r\"IDS0432_220527_RAW_cal__sam_\" ->   <|    \"ζ\" -> 0.000000000000   ,  \"τ1\" -> 0.000000000000   ,  \"τS\" -> 0.000000000000   ,  \"τN\" -> 0.000000000000   ,  \"τC\" -> 0.000000000000   ,  \"κ0\" -> 0.000000000000   ,  \"mm1\" -> 0.000000000000   ,  \"mm2\" -> 0.000000000000   ,  \"mm3\" -> 0.000000000000   ,  \"T\" -> 0.170000000000   ,  \"B\" -> 10.000000000000   ,  \"θ\" -> 0.000000000000   ,  \"Reoff\" -> 0.000000000000   ,  \"Imoff\" -> 0.000000000000   ,  \"στ1\" -> 0.000000000000   ,  \"στS\" -> 0.000000000000   ,  \"στN\" -> 0.000000000000   ,  \"τ11 \" -> 0.000000000000   ,  \"τ12\" -> 0.000000000000   ,  \"τ22\" -> 0.000000000000   ,  \"τN1\" -> 0.000000000000   ,  \"τN2\" -> 0.000000000000   ,  \"σηlogτ1 \" -> 0.000000000000   ,  \"σηlogτS\" -> 0.000000000000   ,  \"σηlogτN\" -> 0.000000000000   ,  \"σlogτ1\" -> 0.000000000000   ,  \"σlogτS\" -> 0.000000000000   ,  \"σlogτN\" -> 0.000000000000   ,  \"σητ1\" -> 0.000000000000   ,  \"σητS \" -> 0.000000000000   ,  \"σητN\" -> 0.000000000000    |>   , \r\"IDS0433_220527_RAW_cal__ref_\" ->   <|    \"ζ\" -> 0.036182096392   ,  \"τ1\" -> 0.021229443945   ,  \"τS\" -> 0.040815710128   ,  \"τN\" -> 0.001336208179   ,  \"τC\" -> 0.001738942563   ,  \"κ0\" -> 0.000000003571   ,  \"mm1\" -> 0.000058400724   ,  \"mm2\" -> 0.020067332674   ,  \"mm3\" -> 0.046519716188   ,  \"T\" -> 0.620000000000   ,  \"B\" -> 10.000000000000   ,  \"θ\" -> 0.000000000000   ,  \"Reoff\" -> -1959183.673469394450   ,  \"Imoff\" -> 0.000000000000   ,  \"στ1\" -> 0.002741018217   ,  \"στS\" -> 0.000061676101   ,  \"στN\" -> 0.001584213819   ,  \"τ11 \" -> 0.000000000000   ,  \"τ12\" -> 0.000000000000   ,  \"τ22\" -> 0.000000000000   ,  \"τN1\" -> 0.000000000000   ,  \"τN2\" -> 0.000000000000   ,  \"σηlogτ1 \" -> 0.000000000000   ,  \"σηlogτS\" -> 0.000000000000   ,  \"σηlogτN\" -> 0.000000000000   ,  \"σlogτ1\" -> 0.000000000000   ,  \"σlogτS\" -> 0.000000000000   ,  \"σlogτN\" -> 0.000000000000   ,  \"σητ1\" -> 0.000000000000   ,  \"σητS \" -> 0.000000000000   ,  \"σητN\" -> 0.000000000000    |>   , \r\"IDS0433_220527_RAW_cal__sam_\" ->   <|    \"ζ\" -> 0.000000000000   ,  \"τ1\" -> 0.000000000000   ,  \"τS\" -> 0.000000000000   ,  \"τN\" -> 0.000000000000   ,  \"τC\" -> 0.000000000000   ,  \"κ0\" -> 0.000000000000   ,  \"mm1\" -> 0.000000000000   ,  \"mm2\" -> 0.000000000000   ,  \"mm3\" -> 0.000000000000   ,  \"T\" -> 0.620000000000   ,  \"B\" -> 10.000000000000   ,  \"θ\" -> 0.000000000000   ,  \"Reoff\" -> 0.000000000000   ,  \"Imoff\" -> 0.000000000000   ,  \"στ1\" -> 
